vi "FTW-JSON-LexicalScan-Whitespace.vi"(0 "JSON String":T1, 11 "error in":errorcluster) -> (4 "JSON String Out":T1, 15 "error out":errorcluster)   [LabVIEW 2015]
uses:
  FTW-JSON-LexicalScan.ctl
panel:
  # "Inputs"
  # "Outputs"
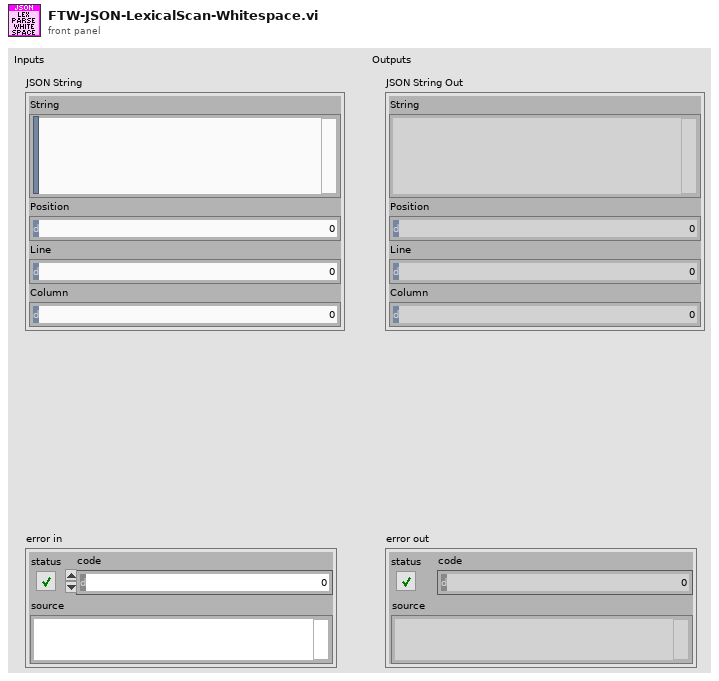
[diagram p1: front panel]
types:
  T1 = typedef "FTW-JSON-LexicalScan.ctl" = cluster{"String":string, "Position":i32, "Line":i32, "Column":i32}
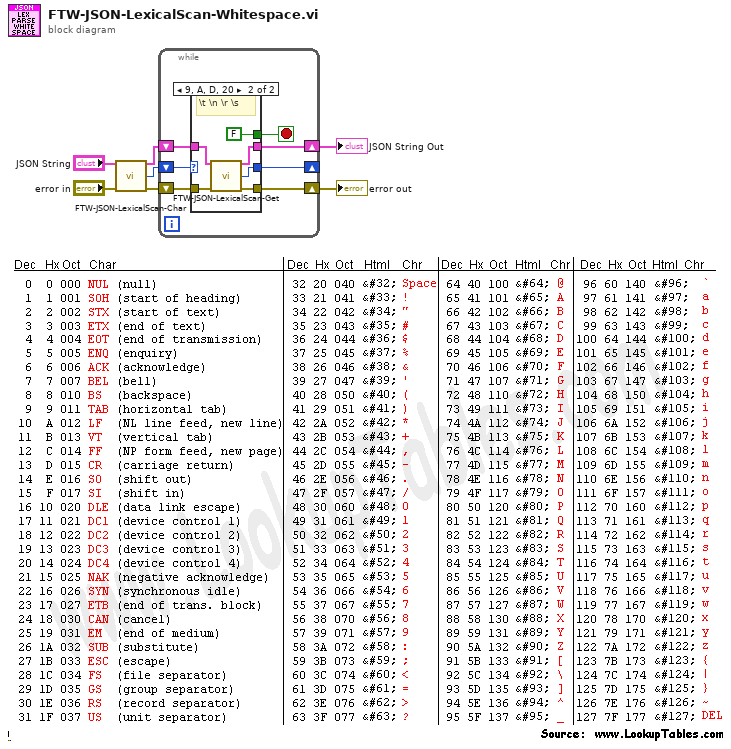
[diagram p0: block diagram]
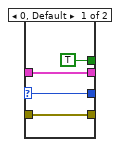
[diagram p2: hidden frame]
diagram:
  n1 = call "FTW-JSON-LexicalScan-Char.vi"("JSON String"="JSON String", "error in"="error in") -> ("JSON String Out"=w2:T1, "Char"=w1:u8, "error out"=w4:errorcluster)  [unwired: 11 in]
  n2 = while {
    shift-right: [w13] -> w6
    shift-left: w2 -> [w11]
    shift-right: [w12] -> w5
    shift-left: w4 -> [w10]
    shift-right: [w8] -> _
    shift-left: w1 -> [w9]
    stop <- w14 stop-if-true
    n3 = case shown="9, A, D, 20" w9 {
      selector: w9 -> [w15 _]
      tunnel: [TRUE FALSE] -> w14
      tunnel: [w17 w20] -> w13
      tunnel: w11 -> [w17 w21]
      tunnel: [w16 w22] -> w12
      tunnel: w10 -> [w16 w23]
      tunnel: [w15 w19] -> w8
      frame 0, Default {
      }
      frame 9, 10, 13, 32 {
        # "\\t \\n \\r \\s"
        n4 = call "FTW-JSON-LexicalScan-Get.vi"("JSON String"=w21, "error in"=w23) -> ("JSON String Out"=w20:T1, "Char"=w19:u8, "error out"=w22:errorcluster)  [unwired: 11 in]
      }
    }
  }
  "error out" <- w5
  "JSON String Out" <- w6
